vi "Get Control Image or Terminal Image to File(冲突时的文件备份2013-05-03 10-53-15).vi"(6 "选择文件类型":enum16{"PNG", "JPG", "BMP"}(ring), 7 "图片文件存储路径":path, 8 "错误输入（无错误）":errorcluster, 9 "类型":enum16{"控件", "接线端"}(ring), 10 "图像参数":cluster{"图像深度":i32, "背景颜色":u32}={"图像深度"=8, "背景颜色"=0} {"图像深度" items=["1位、黑白"=1, "4位、16色"=4, "8位、256色"=8, "24位、真彩色"=24]}, 11 "Ctl Ref In":refnum<vi>) -> (0 "错误输出":errorcluster, 3 "Ctl Ref Out":refnum<vi>)   [LabVIEW 2012, in "CtrlRef.lvlib"]
uses:
  CtrlRef.lvlib
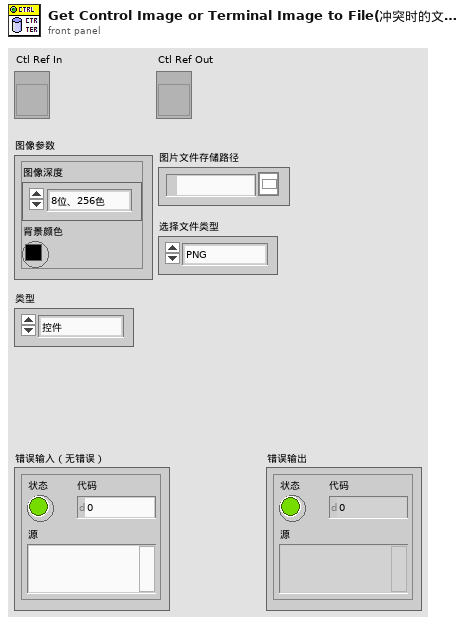
[diagram p1: front panel]
types:
  T1 = typedef "imagedata.ctl" = cluster{"image type":i32, "image depth":i32, "image":u8[], "mask":u8[], "colors":u32[], "Rectangle":cluster{"left":i16, "top":i16, "right":i16, "bottom":i16}}
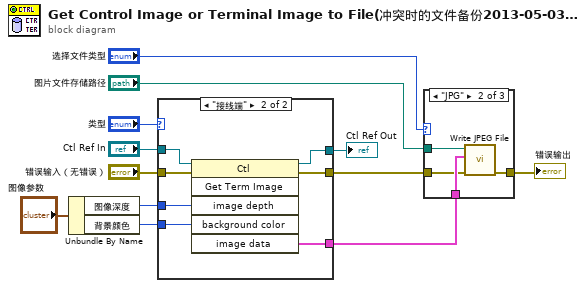
[diagram p0: block diagram]
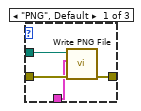
[diagram p2: hidden frame]
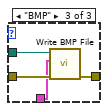
[diagram p3: hidden frame]
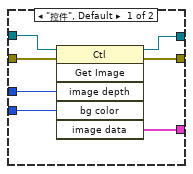
[diagram p4: hidden frame]
diagram:
  n1 = Unbundle By Name("图像参数") -> ("图像深度"=w2:i32, "背景颜色"=w1:u32)
  n2 = case shown="\"接线端\"" "类型" {
    tunnel: "Ctl Ref In" -> [w19 w26]
    tunnel: [w15 w25] -> w10
    tunnel: "错误输入（无错误）" -> [w16 w24]
    tunnel: [w13 w23] -> w5
    tunnel: [w14 w22] -> w7
    tunnel: w2 -> [w18 w21]
    tunnel: w1 -> [w17 w20]
    frame "控件", Default {
      n3 = invoke class="Ctl" method="Get Image"(reference=w19, error in=w16, "image depth"=w18, "bg color"=w17) -> (reference out=w15:refnum<vi>, error out=w13:errorcluster, "image data"=w14:T1)  [unwired: 2 in, 3 out]
    }
    frame "接线端" {
      n4 = invoke class="Ctl" method="Get Term Image"(reference=w26, error in=w24, "image depth"=w21, "background color"=w20) -> (reference out=w25:refnum<vi>, error out=w23:errorcluster, "image data"=w22:T1)  [unwired: 2 in, 3 out]
    }
  }
  "Ctl Ref Out" <- w10
  n5 = case shown="\"JPG\"" "选择文件类型" {
    tunnel: "图片文件存储路径" -> [w27 w31 w36]
    tunnel: w7 -> [w28 w34 w35]
    tunnel: w5 -> [w30 w33 w38]
    tunnel: [w29 w32 w37] -> w4
    frame "PNG", Default {
      n6 = call <vilib>:"Write PNG File.vi"("error in (no error)"=w30, "image data"=w28, "path to PNG file"=w27) -> ("error out"=w29:errorcluster)  [unwired: 7 in, 1 out]
    }
    frame "JPG" {
      n7 = call <vilib>:"Write JPEG File.vi"("error in (no error)"=w33, "image data"=w34, "path to JPEG file"=w31) -> ("error out"=w32:errorcluster)  [unwired: 7 in, 1 out]
    }
    frame "BMP" {
      n8 = call <vilib>:"Write BMP File.vi"("error in (no error)"=w38, "image data"=w35, "path to BMP file"=w36) -> ("error out"=w37:errorcluster)  [unwired: 7 in, 1 out]
    }
  }
  "错误输出" <- w4
